vi "calc_s21.vi"(8 "complex value+1":dbl[](array[numeric]), 9 "complex value":dbl[](array[numeric]), 10 "frequency+1":dbl, 11 "frequency":dbl) -> (3 "s21_data":T1)   [LabVIEW 2025]
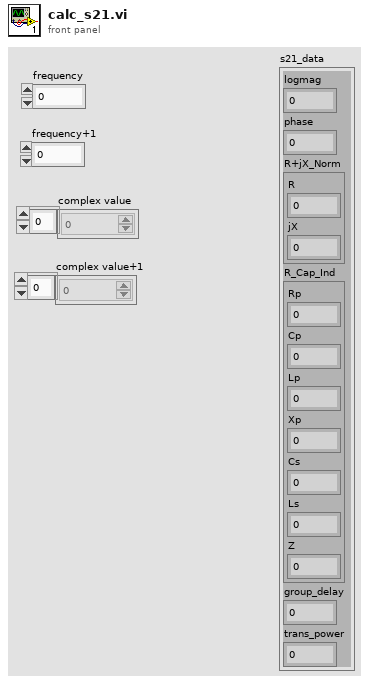
[diagram p1: front panel]
types:
  T1 = cluster{"logmag":dbl, "phase":dbl, "R+jX_Norm":cluster{"R":dbl, "jX":dbl}, "R_Cap_Ind":cluster{"Rp":dbl, "Cp":dbl, "Lp":dbl, "Xp":dbl, "Cs":dbl, "Ls":dbl, "Z":dbl}, "group_delay":dbl, "trans_power":dbl}
  T2 = cluster{"Rp":dbl, "Cp":dbl, "Lp":dbl, "Xp":dbl, "Cs":dbl, "Ls":dbl, "Z":dbl}
  T3 = cluster{"logmag":dbl, "phase":dbl, "R+jX_Norm":cluster{"R":dbl, "jX":dbl}, "R_Cap_Ind":cluster{"Rp":dbl, "Cp":dbl, "Lp":dbl, "Xp":dbl, "Cs":dbl, "Ls":dbl, "Z":dbl}, "group_delay":dbl, "power":dbl}
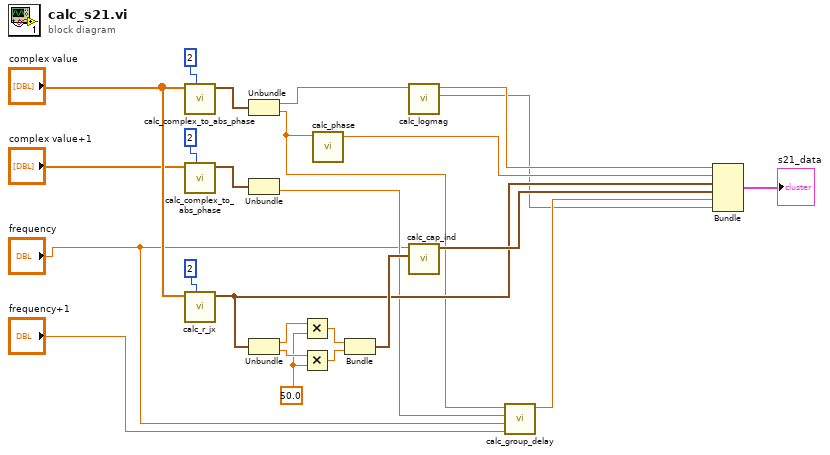
[diagram p0: block diagram]
diagram:
  w19 = 50.0 ("y")
  n1 = call "calc_complex_to_abs_phase.vi"("index"=2, "complex value"="complex value") -> ("output"=w24:cluster{"abs":dbl, "phase":dbl})  [unwired: 9 in]
  n2 = call "calc_complex_to_abs_phase.vi"("index"=2, "complex value"="complex value+1") -> ("output"=w13:cluster{"abs":dbl, "phase":dbl})  [unwired: 9 in]
  n3 = call "calc_r_jx.vi"("index"=2, "complex value"="complex value") -> ("R+jX_Norm"=w14:cluster{"R":dbl, "jX":dbl})  [unwired: 9 in]
  n4 = Unbundle(w24) -> ("abs"=w23:dbl, "phase"=w8:dbl)
  n5 = Unbundle(w13) -> ("phase"=w9:dbl)  [unwired: 1 out]
  n6 = Unbundle(w14) -> ("R"=w21:dbl, "jX"=w20:dbl)
  n7 = Multiply(x=w21, y=w19) -> (x*y=w18:dbl)
  n8 = Multiply(x=w20, y=w19) -> (x*y=w17:dbl)
  n9 = call "calc_phase.vi"("phase [rad]"=w8) -> ("phase"=w10:dbl)  [unwired: 10 in]
  n10 = Bundle(w18, w17) -> (w16:cluster{dbl, dbl})  [unwired: 1 in]
  n11 = call "calc_logmag.vi"("abs"=w23) -> ("power"=w2:dbl, "logmag"=w22:dbl)  [unwired: 9 in]
  n12 = call "calc_cap_ind.vi"("R+jX"=w16, "freq"="frequency") -> ("R_Cap_Ind"=w15:T2)  [unwired: 9 in]
  n13 = call "calc_group_delay.vi"("frequency+1"="frequency+1", "frequency"="frequency", "phase+1"=w9, "phase"=w8) -> ("group_delay"=w11:dbl)  [unwired: 7 in]
  n14 = Bundle("logmag"=w22, "phase"=w10, "R+jX_Norm"=w14, "R_Cap_Ind"=w15, "group_delay"=w11, "power"=w2) -> (→"s21_data":T3)  [unwired: 1 in]
